vi "Begin.vi"(8 "error in":errorcluster) -> (0 "error out":errorcluster)   [LabVIEW 2020]
doc: "Called before other user functions, this VI is expected to open initial I/O refnums, load in file data, and do all program initialization. Notice that the <B>error out</B> terminal is simply used for data flow. Wiring it to other structures or subVIs ensures that this VI runs first."
uses:
  <vilib>/Rock Robotics/WPI/ThirdParty/Phoenix-LabVIEW/Pigeon2/controls/CTRE_Phoenix_Pigeon2_Configurables.ctl
  <vilib>/Rock Robotics/WPI/DriverStation/WPI_DriverStationRobotMode2.ctl
  <vilib>/Rock Robotics/WPI/Joystick/WPI_JoystickDeviceEnum.ctl
  <vilib>/Rock Robotics/SystemInterfaces/i2clib/i2c_bus.ctl
  <vilib>/Rock Robotics/WPI/Solenoid/WPI_SolenoidChannel.ctl
  <vilib>/Rock Robotics/SystemInterfaces/DIO/FPGA_DIOChannel.ctl
  Robot Global Data.vi
  <vilib>/Rock Robotics/Network Tables/NT Write String Array.vi
  <vilib>/Rock Robotics/WPI/Utilities/WPI_GetSetVariantRefNum.vi
  <vilib>/Rock Robotics/WPI/Solenoid/WPI_SolenoidOpenDouble.vi
  <vilib>/Rock Robotics/WPI/ThirdParty/Phoenix-LabVIEW/Motor Controller/Get/CTRE_Phoenix_MotorController_GetSelectedSensorData.vi
  <vilib>/Rock Robotics/WPI/Switch/WPI_SwitchOpenLimit.vi
  <vilib>/Rock Robotics/WPI/Switch/WPI_SwitchOpenCounting.vi
panel:
  in  "Pigeon2 Configurables":T1
  # "Yaw Angle needed to reach the current orientation in degrees"
  # "Configures the mounting pose of the Pigeon2\nThis is the yaw-pitch-roll teh Pigeon2 underwent to get to its current orientation,\n referenced from the robot's point of view\nThis is only necessary if the Pigeon2 is mounted at an exotic angle near the gimbal lock point or not forward.\nIf the pigeon is relatively flat and pointed forward, this is not needed"
  # "Pitch Angle needed to reach the current orientation in degrees"
  # "Roll Angle needed to reach the current orientation in degrees"
  # "Disables the temperature compensation\nfrom the Pigeon2. It is recommended that\nthis remains false"
  # "Disables the no-motion calibration from the\nPigeon2. It is recommended that this \nremains false"
  # "Enables the compass for Pigeon2\nThis is not recommended for any indoor robotics"
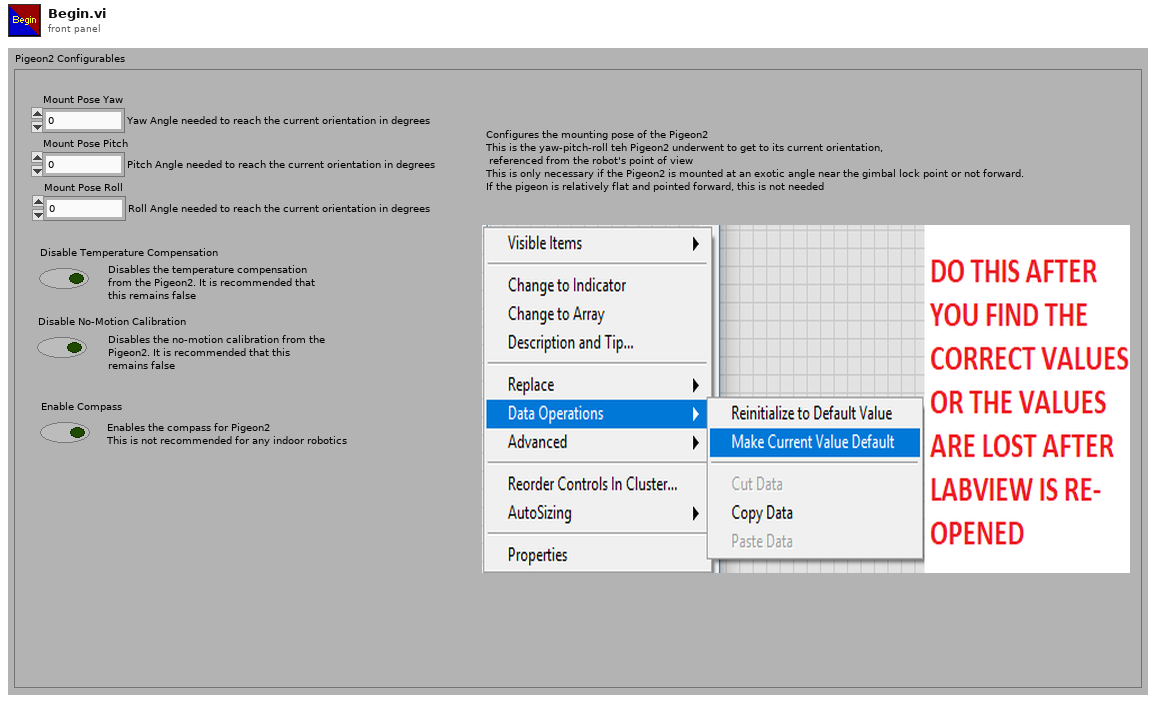
[diagram p1: front panel]
types:
  T1 = typedef "CTRE_Phoenix_Pigeon2_Configurables.ctl" = cluster{"Mount Pose Yaw":dbl, "Mount Pose Pitch":dbl, "Mount Pose Roll":dbl, "Disable Temperature Compensation":bool, "Disable No-Motion Calibration":bool, "Enable Compass":bool}
  T2 = typedef "FPGA_DIOChannel.ctl" = enum8{"DIO 0", "DIO 1", "DIO 2", "DIO 3", "DIO 4", "DIO 5", "DIO 6", "DIO 7", "DIO 8", "DIO 9", "DIO MXP 0", "DIO MXP 1", "DIO MXP 2", "DIO MXP 3", "DIO MXP 4", "DIO MXP 5", "DIO MXP 6", "DIO MXP 7", "DIO MXP 8", "DIO MXP 9", "DIO MXP 10", "DIO MXP 11", "DIO MXP 12", "DIO MXP 13", "DIO MXP 14", "DIO MXP 15", "SPI Port CS1", "SPI Port CS2", "SPI Port CS3", "SPI Port MISO", "SPI Port MOSI", "Invalid"}
  T3 = typedef "WPI_SolenoidChannel.ctl" = enum8{"Solenoid 0", "Solenoid 1", "Solenoid 2", "Solenoid 3", "Solenoid 4", "Solenoid 5", "Solenoid 6", "Solenoid 7", "Solenoid 8", "Solenoid 9", "Solenoid 10", "Solenoid 11", "Solenoid 12", "Solenoid 13", "Solenoid 14", "Solenoid 15", "Invalid"}
  T4 = typedef "i2c_bus.ctl" = enum16{"I2C On-Board", "I2C MXP", "Invalid"}
  T5 = typedef "WPI_JoystickDeviceEnum.ctl" = enum16{"USB 0", "USB 1", "USB 2", "USB 3", "USB 4", "USB 5"}
  T6 = typedef "WPI_DriverStationRobotMode2.ctl" = enum16{"Autonomous Disabled", "Autonomous Enabled", "Teleop Disabled", "Teleop Enabled", "Disconnected", "Finish", "Test Disabled", "Test Enabled", "Emergency Stopped"}
  T7 = typedef "WPI_JoystickDevRef.ctl" = cluster{"Device":T5}
  T8 = typedef "WPI_SolenoidDevRef.ctl" = cluster{"DevStatus":errorcluster, "Pneumatics Control Module":u8, "Forward Solenoid Channel":T3, "Reverse Solenoid Channel":T3}
  T9 = typedef "WPI_CompressorDevRef.ctl" = cluster{"DevStatus":errorcluster, "Pneumatics Control Module":u8}
  T10 = typedef "WPI_SwitchDevRef.ctl" = cluster{"DevStatus":errorcluster, "DIO Channel":T2, "CntIndex":T11, "Normally Closed":bool}
  T11 = typedef "FPGA_CounterCtrSystemIndex.ctl" = enum8{"Ctr 0", "Ctr 1", "Ctr 2", "Ctr 3", "Ctr 4", "Ctr 5", "Ctr 6", "Ctr 7", "Invalid"}
  T12 = typedef "WPI_MotorControlDeviceRef.ctl" = cluster{"DeviceStatus":errorcluster, "Type":T13, "PWM":cluster{"PWM Channel":T14, "DeadBand":T15}, "CAN":cluster{"Device Number":u8, "SetOutput VI Ref":variant, "GetOutput VI Ref":variant, "Enable VI Ref":variant, "Disable VI Ref":variant, "Data":variant}, "Invert":bool, "DIO PWM":cluster{"PWM \"Enable\" Channel":T14, "DIOChannel":T2, "PWM Rate":dbl}}
  T13 = typedef "WPI_MotorControlType.ctl" = enum16{"PWM", "CAN", "DIO PWM"}
  T14 = typedef "FPGA_DIOPWMChannel.ctl" = enum8{"PWM 0", "PWM 1", "PWM 2", "PWM 3", "PWM 4", "PWM 5", "PWM 6", "PWM 7", "PWM 8", "PWM 9", "PWM MXP 0", "PWM MXP 1", "PWM MXP 2", "PWM MXP 3", "PWM MXP 4", "PWM MXP 5", "PWM MXP 6", "PWM MXP 7", "PWM MXP 8", "PWM MXP 9", "Invalid"}
  T15 = typedef "WPI_PWMDeadband.ctl" = cluster{"Name":string, "maxPositivePwm":i32, "minPositivePwm":i32, "centerPwm":i32, "maxNegativePwm":i32, "minNegativePwm":i32, "angularRange":u16}
  T16 = typedef "Color Sensor V3 DevRef.ctl" = cluster{"I2CDevRef":T17}
  T17 = typedef "WPI_I2CDevRef.ctl" = cluster{"DevStatus":errorcluster, "Device Address":u8, "Handle":i32, "I2C Bus":T4}
  T18 = typedef "CTRE_Phoenix_CANcoder_DeviceRef.ctl" = cluster{"DeviceStatus":errorcluster, "Device Number":u8, "Handle":u64, "UsageFrame":u32, "Library Path":path}
  T19 = typedef "CTRE_PigeonIMU_DeviceRef.ctl" = cluster{"DeviceStatus":errorcluster, "Device Number":u8, "Type":T20, "Device ID":u32, "Handle":u64, "UsageFrame":u32, "Library Path":path}
  T20 = typedef "CTRE_PigeonIMU_ConnectionType.ctl" = u32
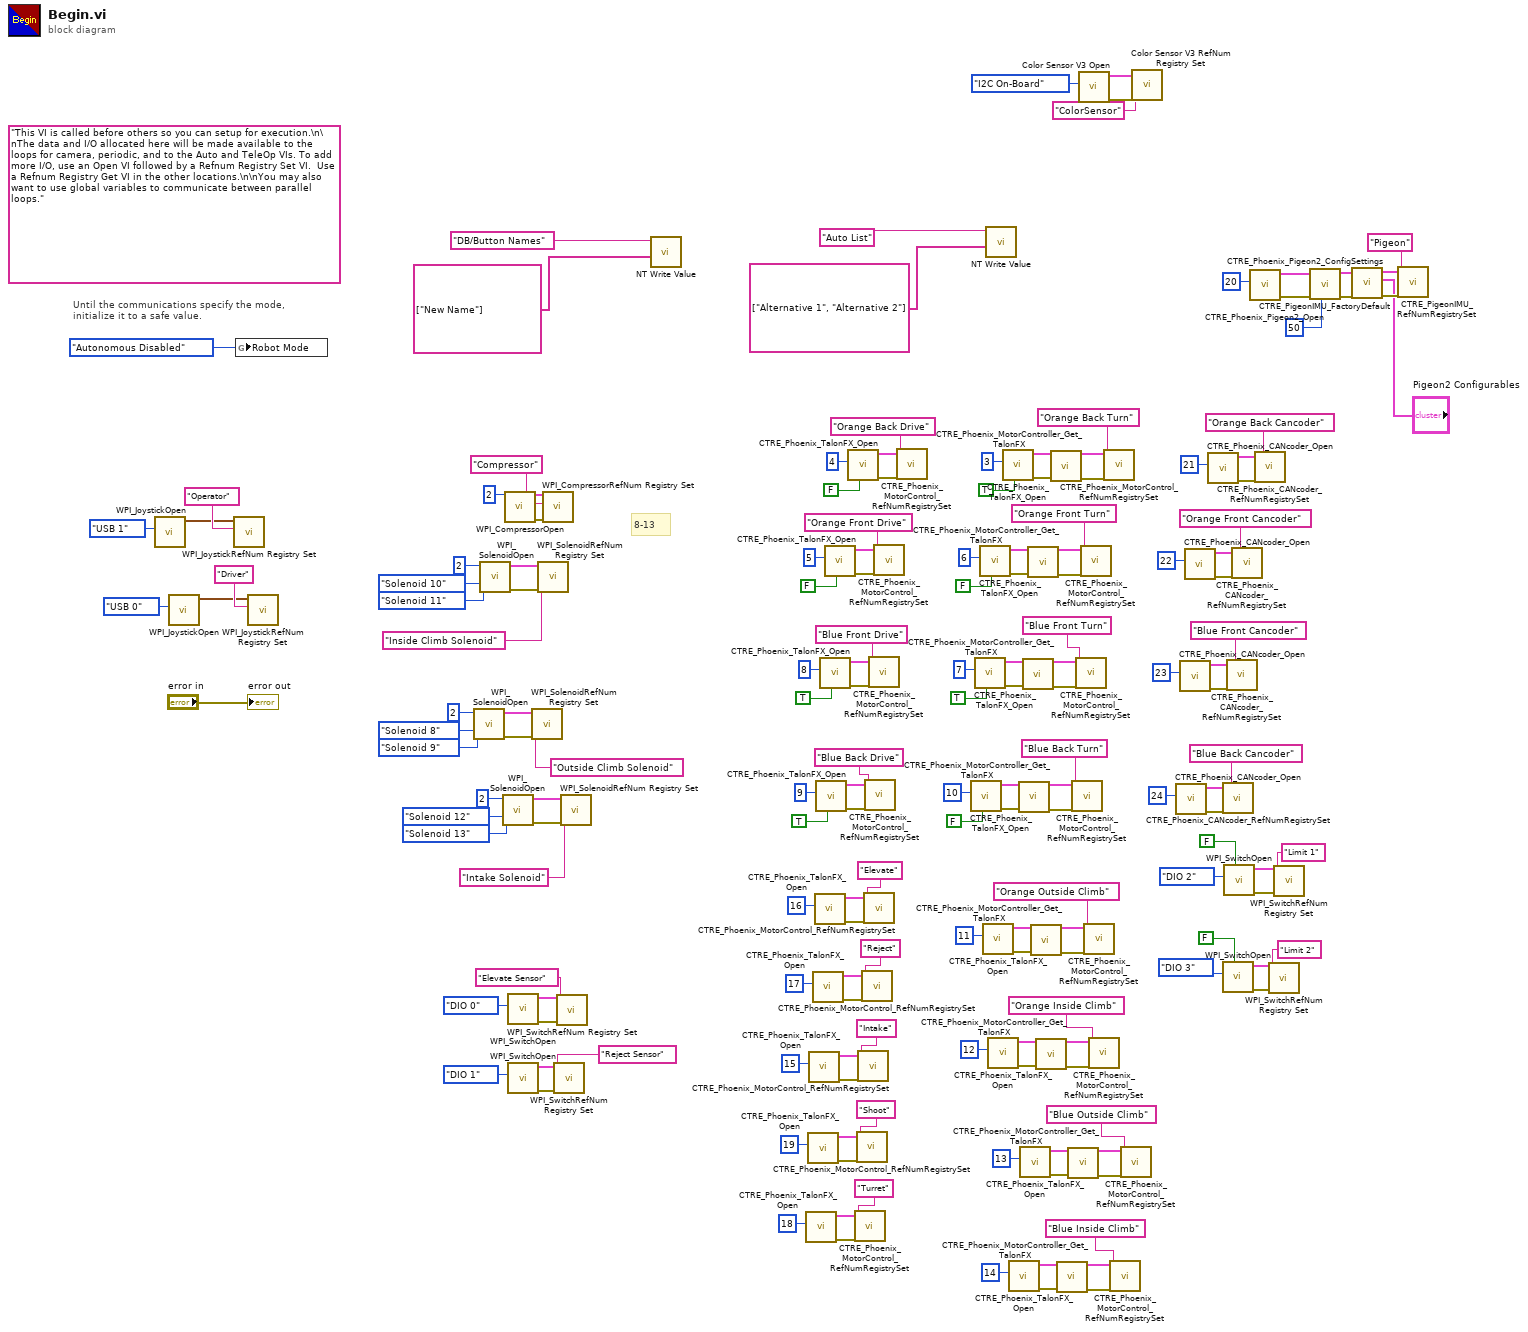
[diagram p0: block diagram]
diagram:
  (unwired) "This VI is called before others so you can setup for execution.\n\nThe data and I/O allocated here will be made available to the loops for camera, periodic, and to the Auto and TeleOp VIs. To add more I/O, use an Open VI followed by a Refnum Registry Set VI.  Use a Refnum Registry Get VI in the other locations.\n\nYou may also want to use global variables to communicate between parallel loops."
  # "8-13"
  # "Until the communications specify the mode,\ninitialize it to a safe value."
  n1 = call <vilib>:"WPI_JoystickOpen.vi"("JoystickDevice"=WPI_JoystickDeviceEnum."USB 1") -> ("JoystickDevRef"=w164:T7)  [unwired: 10 in]
  n2 = call <vilib>:"WPI_JoystickOpen.vi"("JoystickDevice"=WPI_JoystickDeviceEnum."USB 0") -> ("JoystickDevRef"=w172:T7)  [unwired: 10 in]
  n3 = call <vilib>:"WPI_JoystickRefNum Registry Set.vi"("refnum name"="Operator", "JoystickDevRef"=w164) -> ()  [unwired: 8 in, 2 out]
  n4 = global write "Robot Global Data.vi" "Robot Mode"(WPI_DriverStationRobotMode2."Autonomous Disabled" ("Robot Mode")) -> ()
  n5 = call <vilib>:"WPI_JoystickRefNum Registry Set.vi"("refnum name"="Driver", "JoystickDevRef"=w172) -> ()  [unwired: 8 in, 2 out]
  n6 = call-poly <vilib>:"WPI_SolenoidOpen.vi"("Reverse Solenoid Channel"=WPI_SolenoidChannel."Solenoid 9", "Forward Solenoid Channel"=WPI_SolenoidChannel."Solenoid 8", "Pneumatics Device (def)"=u8 2) -> ("error out"=w74:errorcluster, "SolenoidDevRef"=w73:T8)  [unwired: 7 in]
  n7 = call-poly <vilib>:"WPI_SolenoidOpen.vi"("Reverse Solenoid Channel"=WPI_SolenoidChannel."Solenoid 11", "Forward Solenoid Channel"=WPI_SolenoidChannel."Solenoid 10", "Pneumatics Device (def)"=u8 2) -> ("error out"=w77:errorcluster, "SolenoidDevRef"=w76:T8)  [unwired: 7 in]
  n8 = call-poly <vilib>:"WPI_SolenoidOpen.vi"("Reverse Solenoid Channel"=WPI_SolenoidChannel."Solenoid 13", "Forward Solenoid Channel"=WPI_SolenoidChannel."Solenoid 12", "Pneumatics Device (def)"=u8 2) -> ("error out"=w71:errorcluster, "SolenoidDevRef"=w70:T8)  [unwired: 7 in]
  n9 = call <vilib>:"WPI_CompressorOpen.vi"("Pneumatics device (def)"=u8 2) -> ("CompressorDevRef"=w80:T9, "error out"=w81:errorcluster)  [unwired: 13 in]
  n10 = call-poly <vilib>:"WPI_SwitchOpen.vi"("DIO Channel"=FPGA_DIOChannel."DIO 0") -> ("error out"=w35:errorcluster, "SwitchDevRef"=w34:T10)  [unwired: 9 in]
  n11 = call-poly <vilib>:"WPI_SwitchOpen.vi"("DIO Channel"=FPGA_DIOChannel."DIO 1") -> ("error out"=w31:errorcluster, "SwitchDevRef"=w30:T10)  [unwired: 9 in]
  n12 = call <vilib>:"WPI_SolenoidRefNum Registry Set.vi"("error in (no error)"=w74, "refnum name"="Outside Climb Solenoid", "SolenoidDevRef"=w73) -> ()  [unwired: 7 in, 2 out]
  n13 = call <vilib>:"WPI_SolenoidRefNum Registry Set.vi"("error in (no error)"=w77, "refnum name"="Inside Climb Solenoid", "SolenoidDevRef"=w76) -> ()  [unwired: 7 in, 2 out]
  n14 = call <vilib>:"WPI_CompressorRefNum Registry Set.vi"("error in (no error)"=w81, "refnum name"="Compressor", "CompressorDevRef"=w80) -> ()  [unwired: 7 in, 2 out]
  n15 = call <vilib>:"WPI_SwitchRefNum Registry Set.vi"("error in (no error)"=w31, "refnum name"="Reject Sensor", "SwitchDevRef"=w30) -> ()  [unwired: 7 in, 2 out]
  n16 = call <vilib>:"WPI_SwitchRefNum Registry Set.vi"("error in (no error)"=w35, "refnum name"="Elevate Sensor", "SwitchDevRef"=w34) -> ()  [unwired: 7 in, 2 out]
  n17 = call <vilib>:"WPI_SolenoidRefNum Registry Set.vi"("error in (no error)"=w71, "refnum name"="Intake Solenoid", "SolenoidDevRef"=w70) -> ()  [unwired: 7 in, 2 out]
  n18 = call-poly <vilib>:"NT Write Value.vi"("String Array"=string[] ["New Name"], "Name"="DB/Button Names") -> ()  [unwired: 9 in, 1 out]
  n19 = call <vilib>:"CTRE_Phoenix_TalonFX_Open.vi"("Device Number"=u8 18) -> ("error out"=w89:errorcluster, "PhoenixMotorControlDevRef"=w88:T12)  [unwired: 9 in]
  n20 = call <vilib>:"CTRE_Phoenix_TalonFX_Open.vi"("Device Number"=u8 19) -> ("error out"=w93:errorcluster, "PhoenixMotorControlDevRef"=w92:T12)  [unwired: 9 in]
  n21 = call <vilib>:"CTRE_Phoenix_TalonFX_Open.vi"("Device Number"=u8 15) -> ("error out"=w101:errorcluster, "PhoenixMotorControlDevRef"=w100:T12)  [unwired: 9 in]
  n22 = call <vilib>:"CTRE_Phoenix_TalonFX_Open.vi"("Device Number"=u8 17) -> ("error out"=w97:errorcluster, "PhoenixMotorControlDevRef"=w96:T12)  [unwired: 9 in]
  n23 = call <vilib>:"CTRE_Phoenix_TalonFX_Open.vi"("Device Number"=u8 16) -> ("error out"=w105:errorcluster, "PhoenixMotorControlDevRef"=w104:T12)  [unwired: 9 in]
  n24 = call <vilib>:"CTRE_Phoenix_TalonFX_Open.vi"("Invert"=TRUE, "Device Number"=u8 9) -> ("error out"=w119:errorcluster, "PhoenixMotorControlDevRef"=w118:T12)  [unwired: 8 in]
  n25 = call <vilib>:"CTRE_Phoenix_TalonFX_Open.vi"("Invert"=TRUE, "Device Number"=u8 8) -> ("error out"=w133:errorcluster, "PhoenixMotorControlDevRef"=w132:T12)  [unwired: 8 in]
  n26 = call <vilib>:"CTRE_Phoenix_TalonFX_Open.vi"("Invert"=FALSE, "Device Number"=u8 5) -> ("error out"=w147:errorcluster, "PhoenixMotorControlDevRef"=w146:T12)  [unwired: 8 in]
  n27 = call <vilib>:"CTRE_Phoenix_TalonFX_Open.vi"("Invert"=FALSE, "Device Number"=u8 4) -> ("error out"=w162:errorcluster, "PhoenixMotorControlDevRef"=w161:T12)  [unwired: 8 in]
  n28 = call <vilib>:"CTRE_Phoenix_MotorControl_RefNumRegistrySet.vi"("error in (no error)"=w89, "refnum name"="Turret", "PhoenixMotorControlDevRef"=w88) -> ()  [unwired: 7 in, 2 out]
  n29 = call <vilib>:"CTRE_Phoenix_MotorControl_RefNumRegistrySet.vi"("error in (no error)"=w93, "refnum name"="Shoot", "PhoenixMotorControlDevRef"=w92) -> ()  [unwired: 7 in, 2 out]
  n30 = call <vilib>:"CTRE_Phoenix_MotorControl_RefNumRegistrySet.vi"("error in (no error)"=w101, "refnum name"="Intake", "PhoenixMotorControlDevRef"=w100) -> ()  [unwired: 7 in, 2 out]
  n31 = call <vilib>:"CTRE_Phoenix_MotorControl_RefNumRegistrySet.vi"("error in (no error)"=w97, "refnum name"="Reject", "PhoenixMotorControlDevRef"=w96) -> ()  [unwired: 7 in, 2 out]
  n32 = call <vilib>:"CTRE_Phoenix_MotorControl_RefNumRegistrySet.vi"("error in (no error)"=w105, "refnum name"="Elevate", "PhoenixMotorControlDevRef"=w104) -> ()  [unwired: 7 in, 2 out]
  n33 = call <vilib>:"CTRE_Phoenix_MotorControl_RefNumRegistrySet.vi"("error in (no error)"=w119, "refnum name"="Blue Back Drive", "PhoenixMotorControlDevRef"=w118) -> ()  [unwired: 7 in, 2 out]
  n34 = call <vilib>:"CTRE_Phoenix_MotorControl_RefNumRegistrySet.vi"("error in (no error)"=w133, "refnum name"="Blue Front Drive", "PhoenixMotorControlDevRef"=w132) -> ()  [unwired: 7 in, 2 out]
  n35 = call <vilib>:"CTRE_Phoenix_MotorControl_RefNumRegistrySet.vi"("error in (no error)"=w147, "refnum name"="Orange Front Drive", "PhoenixMotorControlDevRef"=w146) -> ()  [unwired: 7 in, 2 out]
  n36 = call <vilib>:"CTRE_Phoenix_MotorControl_RefNumRegistrySet.vi"("error in (no error)"=w162, "refnum name"="Orange Back Drive", "PhoenixMotorControlDevRef"=w161) -> ()  [unwired: 7 in, 2 out]
  n37 = call <vilib>:"CTRE_Phoenix_TalonFX_Open.vi"("Invert"=FALSE, "Device Number"=u8 10) -> ("error out"=w116:errorcluster, "PhoenixMotorControlDevRef"=w117:T12)  [unwired: 8 in]
  n38 = call <vilib>:"CTRE_Phoenix_TalonFX_Open.vi"("Invert"=TRUE, "Device Number"=u8 7) -> ("error out"=w130:errorcluster, "PhoenixMotorControlDevRef"=w131:T12)  [unwired: 8 in]
  n39 = call <vilib>:"CTRE_Phoenix_TalonFX_Open.vi"("Invert"=FALSE, "Device Number"=u8 6) -> ("error out"=w144:errorcluster, "PhoenixMotorControlDevRef"=w145:T12)  [unwired: 8 in]
  n40 = call <vilib>:"CTRE_Phoenix_TalonFX_Open.vi"("Device Number"=u8 11) -> ("error out"=w58:errorcluster, "PhoenixMotorControlDevRef"=w59:T12)  [unwired: 9 in]
  n41 = call-poly <vilib>:"NT Write Value.vi"("String Array"=string[] ["Alternative 1", "Alternative 2"], "Name"="Auto List") -> ()  [unwired: 9 in, 1 out]
  n42 = call <vilib>:"CTRE_Phoenix_TalonFX_Open.vi"("Device Number"=u8 12) -> ("error out"=w52:errorcluster, "PhoenixMotorControlDevRef"=w53:T12)  [unwired: 9 in]
  n43 = call <vilib>:"CTRE_Phoenix_TalonFX_Open.vi"("Invert"=TRUE, "Device Number"=u8 3) -> ("error out"=w159:errorcluster, "PhoenixMotorControlDevRef"=w160:T12)  [unwired: 8 in]
  n44 = call <vilib>:"CTRE_Phoenix_TalonFX_Open.vi"("Device Number"=u8 14) -> ("error out"=w40:errorcluster, "PhoenixMotorControlDevRef"=w41:T12)  [unwired: 9 in]
  n45 = call-poly <vilib>:"CTRE_Phoenix_MotorController_Get_TalonFX.vi"("PhoenixMotorControlDevRef"=w117, "error in"=w116) -> ("PhoenixMotorControlDevRef"=w114:T12, "error out"=w115:errorcluster)  [unwired: 10 in, 2 out]
  n46 = call <vilib>:"CTRE_Phoenix_TalonFX_Open.vi"("Device Number"=u8 13) -> ("error out"=w46:errorcluster, "PhoenixMotorControlDevRef"=w47:T12)  [unwired: 9 in]
  n47 = call-poly <vilib>:"CTRE_Phoenix_MotorController_Get_TalonFX.vi"("PhoenixMotorControlDevRef"=w131, "error in"=w130) -> ("PhoenixMotorControlDevRef"=w128:T12, "error out"=w129:errorcluster)  [unwired: 10 in, 2 out]
  n48 = call-poly <vilib>:"CTRE_Phoenix_MotorController_Get_TalonFX.vi"("PhoenixMotorControlDevRef"=w145, "error in"=w144) -> ("PhoenixMotorControlDevRef"=w142:T12, "error out"=w143:errorcluster)  [unwired: 10 in, 2 out]
  n49 = call-poly <vilib>:"CTRE_Phoenix_MotorController_Get_TalonFX.vi"("PhoenixMotorControlDevRef"=w59, "error in"=w58) -> ("PhoenixMotorControlDevRef"=w56:T12, "error out"=w57:errorcluster)  [unwired: 10 in, 2 out]
  n50 = call-poly <vilib>:"CTRE_Phoenix_MotorController_Get_TalonFX.vi"("PhoenixMotorControlDevRef"=w53, "error in"=w52) -> ("PhoenixMotorControlDevRef"=w50:T12, "error out"=w51:errorcluster)  [unwired: 10 in, 2 out]
  n51 = call-poly <vilib>:"CTRE_Phoenix_MotorController_Get_TalonFX.vi"("PhoenixMotorControlDevRef"=w160, "error in"=w159) -> ("PhoenixMotorControlDevRef"=w157:T12, "error out"=w158:errorcluster)  [unwired: 10 in, 2 out]
  n52 = call-poly <vilib>:"CTRE_Phoenix_MotorController_Get_TalonFX.vi"("PhoenixMotorControlDevRef"=w41, "error in"=w40) -> ("PhoenixMotorControlDevRef"=w38:T12, "error out"=w39:errorcluster)  [unwired: 10 in, 2 out]
  n53 = call-poly <vilib>:"CTRE_Phoenix_MotorController_Get_TalonFX.vi"("PhoenixMotorControlDevRef"=w47, "error in"=w46) -> ("PhoenixMotorControlDevRef"=w44:T12, "error out"=w45:errorcluster)  [unwired: 10 in, 2 out]
  n54 = call <vilib>:"CTRE_Phoenix_MotorControl_RefNumRegistrySet.vi"("error in (no error)"=w115, "refnum name"="Blue Back Turn", "PhoenixMotorControlDevRef"=w114) -> ()  [unwired: 7 in, 2 out]
  n55 = call <vilib>:"CTRE_Phoenix_MotorControl_RefNumRegistrySet.vi"("error in (no error)"=w129, "refnum name"="Blue Front Turn", "PhoenixMotorControlDevRef"=w128) -> ()  [unwired: 7 in, 2 out]
  n56 = call <vilib>:"Color Sensor V3 Open.vi"("I2C Bus"=i2c_bus."I2C On-Board") -> ("error out"=w85:errorcluster, "ColorSensorDevRef"=w84:T16)  [unwired: 9 in]
  n57 = call <vilib>:"CTRE_Phoenix_MotorControl_RefNumRegistrySet.vi"("error in (no error)"=w143, "refnum name"="Orange Front Turn", "PhoenixMotorControlDevRef"=w142) -> ()  [unwired: 7 in, 2 out]
  n58 = call <vilib>:"CTRE_Phoenix_MotorControl_RefNumRegistrySet.vi"("error in (no error)"=w57, "refnum name"="Orange Outside Climb", "PhoenixMotorControlDevRef"=w56) -> ()  [unwired: 7 in, 2 out]
  n59 = call <vilib>:"CTRE_Phoenix_MotorControl_RefNumRegistrySet.vi"("error in (no error)"=w51, "refnum name"="Orange Inside Climb", "PhoenixMotorControlDevRef"=w50) -> ()  [unwired: 7 in, 2 out]
  n60 = call <vilib>:"CTRE_Phoenix_MotorControl_RefNumRegistrySet.vi"("error in (no error)"=w158, "refnum name"="Orange Back Turn", "PhoenixMotorControlDevRef"=w157) -> ()  [unwired: 7 in, 2 out]
  n61 = call <vilib>:"CTRE_Phoenix_MotorControl_RefNumRegistrySet.vi"("error in (no error)"=w39, "refnum name"="Blue Inside Climb", "PhoenixMotorControlDevRef"=w38) -> ()  [unwired: 7 in, 2 out]
  n62 = call <vilib>:"CTRE_Phoenix_MotorControl_RefNumRegistrySet.vi"("error in (no error)"=w45, "refnum name"="Blue Outside Climb", "PhoenixMotorControlDevRef"=w44) -> ()  [unwired: 7 in, 2 out]
  n63 = call <vilib>:"Color Sensor V3 RefNum Registry Set.vi"("error in (no error)"=w85, "refnum name"="ColorSensor", "ColorSensorDevRef"=w84) -> ()  [unwired: 7 in, 2 out]
  n64 = call <vilib>:"CTRE_Phoenix_CANcoder_Open.vi"("Device Number"=u8 24) -> ("error out"=w113:errorcluster, "CTRE_CANcoder_DeviceRef"=w112:T18)  [unwired: 9 in]
  n65 = call <vilib>:"CTRE_Phoenix_CANcoder_Open.vi"("Device Number"=u8 23) -> ("error out"=w127:errorcluster, "CTRE_CANcoder_DeviceRef"=w126:T18)  [unwired: 9 in]
  n66 = call <vilib>:"CTRE_Phoenix_CANcoder_Open.vi"("Device Number"=u8 22) -> ("error out"=w141:errorcluster, "CTRE_CANcoder_DeviceRef"=w140:T18)  [unwired: 9 in]
  n67 = call <vilib>:"CTRE_Phoenix_CANcoder_Open.vi"("Device Number"=u8 21) -> ("error out"=w156:errorcluster, "CTRE_CANcoder_DeviceRef"=w155:T18)  [unwired: 9 in]
  n68 = call <vilib>:"CTRE_Phoenix_CANcoder_RefNumRegistrySet.vi"("error in (no error)"=w113, "refnum name"="Blue Back Cancoder", "CTRE_CANcoder_DeviceRef"=w112) -> ()  [unwired: 7 in, 2 out]
  n69 = call-poly <vilib>:"WPI_SwitchOpen.vi"("Normally Closed"=FALSE, "DIO Channel"=FPGA_DIOChannel."DIO 3") -> ("error out"=w23:errorcluster, "SwitchDevRef"=w22:T10)  [unwired: 8 in]
  n70 = call-poly <vilib>:"WPI_SwitchOpen.vi"("Normally Closed"=FALSE, "DIO Channel"=FPGA_DIOChannel."DIO 2") -> ("error out"=w20:errorcluster, "SwitchDevRef"=w19:T10)  [unwired: 8 in]
  n71 = call <vilib>:"CTRE_Phoenix_CANcoder_RefNumRegistrySet.vi"("error in (no error)"=w127, "refnum name"="Blue Front Cancoder", "CTRE_CANcoder_DeviceRef"=w126) -> ()  [unwired: 7 in, 2 out]
  n72 = call <vilib>:"CTRE_Phoenix_CANcoder_RefNumRegistrySet.vi"("error in (no error)"=w141, "refnum name"="Orange Front Cancoder", "CTRE_CANcoder_DeviceRef"=w140) -> ()  [unwired: 7 in, 2 out]
  n73 = call <vilib>:"CTRE_Phoenix_Pigeon2_Open.vi"("Device Number"=u8 20) -> ("error out"=w4:errorcluster, "PigeonIMUDevRef"=w5:T19)  [unwired: 9 in]
  n74 = call <vilib>:"CTRE_Phoenix_CANcoder_RefNumRegistrySet.vi"("error in (no error)"=w156, "refnum name"="Orange Back Cancoder", "CTRE_CANcoder_DeviceRef"=w155) -> ()  [unwired: 7 in, 2 out]
  n75 = call <vilib>:"WPI_SwitchRefNum Registry Set.vi"("error in (no error)"=w23, "refnum name"="Limit 2", "SwitchDevRef"=w22) -> ()  [unwired: 7 in, 2 out]
  n76 = call <vilib>:"WPI_SwitchRefNum Registry Set.vi"("error in (no error)"=w20, "refnum name"="Limit 1", "SwitchDevRef"=w19) -> ()  [unwired: 7 in, 2 out]
  n77 = call <vilib>:"CTRE_PigeonIMU_FactoryDefault.vi"("timeoutMs"=50, "error in"=w4, "PigeonIMUDevRef"=w5) -> ("error out"=w9:errorcluster, "PigeonIMUDevRef"=w8:T19)  [unwired: 7 in]
  n78 = call <vilib>:"CTRE_Phoenix_Pigeon2_ConfigSettings.vi"("error in (no error)"=w9, "Pigeon2 Configurables"="Pigeon2 Configurables", "PigeonIMUDevRef 2"=w8) -> ("error out"=w7:errorcluster, "PigeonIMUDevRef"=w6:T19)  [unwired: 7 in]
  n79 = call <vilib>:"CTRE_PigeonIMU_RefNumRegistrySet.vi"("error in (no error)"=w7, "refnum name"="Pigeon", "PigeonIMUDevRef"=w6) -> ()  [unwired: 7 in, 2 out]
  "error out" <- "error in"
